vi "Read Controls from Config File.vi"(6 "Child?":bool, 7 "section":string, 8 "Error In":errorcluster, 9 "ParentName":string, 10 "Ctl Refnum":refnum<vi>, 11 "refnum":T1) -> (0 "Error Out":errorcluster, 3 "refnum out":T1)   [LabVIEW 2018]
uses:
  <vilib>/Utility/config.llb/Config Data RefNum.ctl
  Hardware Mfg/Thorlabs Translation Stages/Controls/Translation Stage Cluster.ctl
  Controls/Translation Stage Types.ctl
  <vilib>/Utility/config.llb/Read Key (String).vi
  <vilib>/Utility/config.llb/Read Key (Boolean).vi
  <vilib>/Utility/config.llb/Read Key (Double).vi
  <vilib>/Utility/config.llb/Read Key (U32).vi
  <vilib>/Utility/config.llb/NI_LVConfig.lvlib
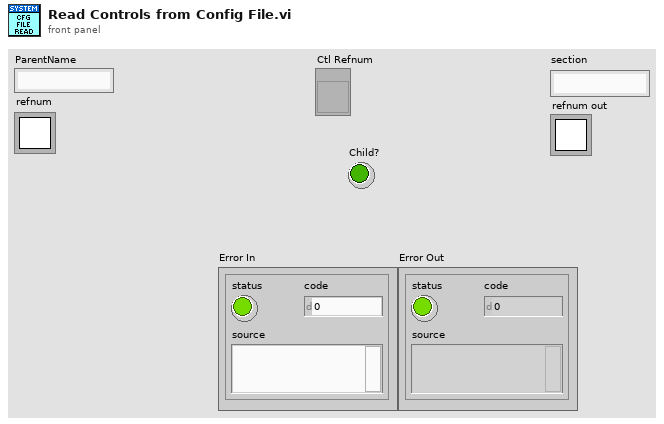
[diagram p1: front panel]
types:
  T1 = typedef "NI_LVConfig.lvlib/Config Data RefNum.ctl" = refnum<k1>
  T2 = typedef "Translation Stage Cluster.ctl" = cluster{"Position":dbl, "Is.Enabled?":bool, "Is.Connected?":bool, "Device SN":string, "AccelerationMaximum":dbl, "VelocityMaximum":dbl, "Acceleration":dbl, "Velocity":dbl, "waitTimeout (ms)":i32, "Model":T3, "Is.Homed?":bool, "MOVE":bool}
  T3 = typedef "Translation Stage Types.ctl" = enum16{"None", "Thorlabs LTS", "Thorlabs MLJ"}
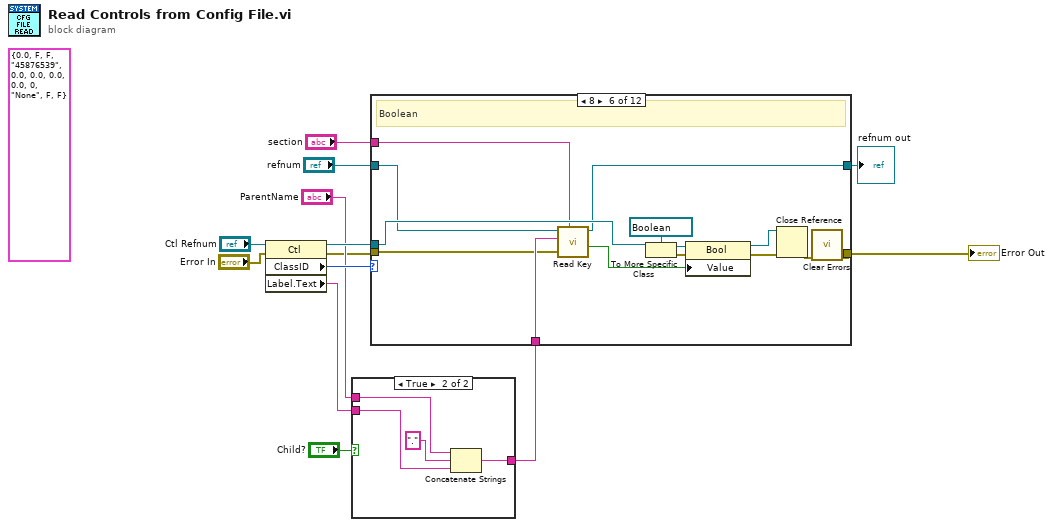
[diagram p0: block diagram]
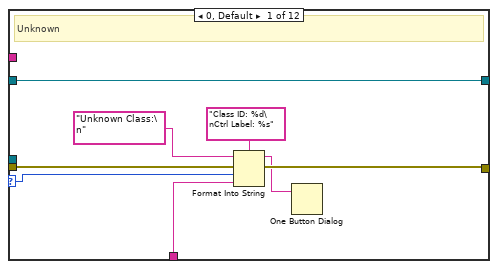
[diagram p3: hidden frame]
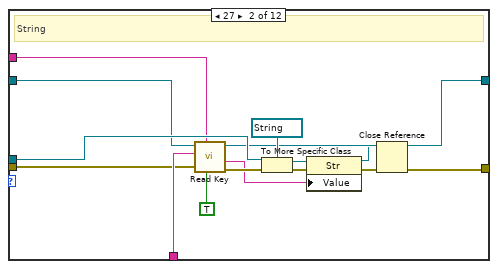
[diagram p4: hidden frame]
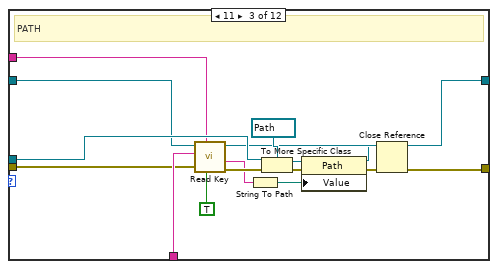
[diagram p5: hidden frame]
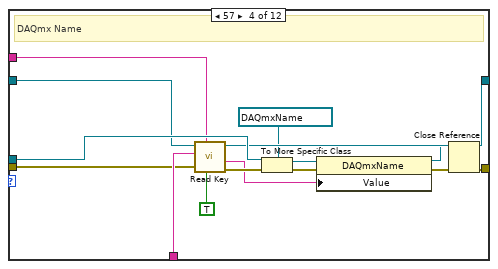
[diagram p6: hidden frame]
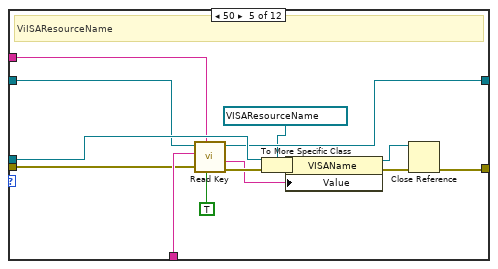
[diagram p7: hidden frame]
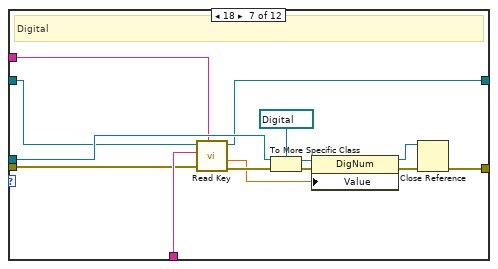
[diagram p8: hidden frame]
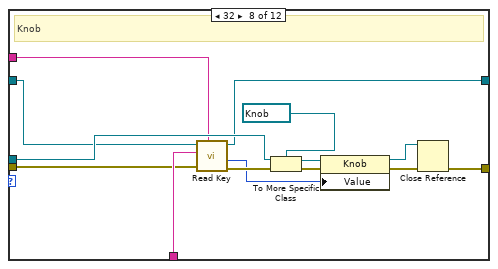
[diagram p9: hidden frame]
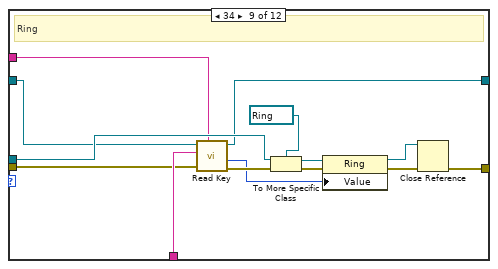
[diagram p10: hidden frame]
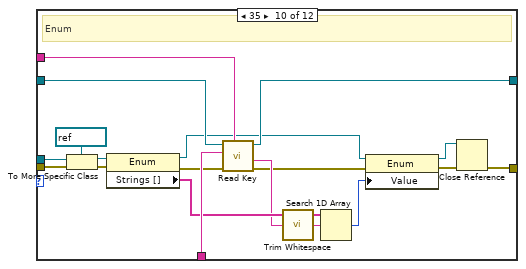
[diagram p11: hidden frame]
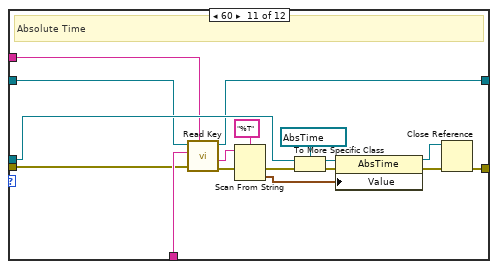
[diagram p12: hidden frame]
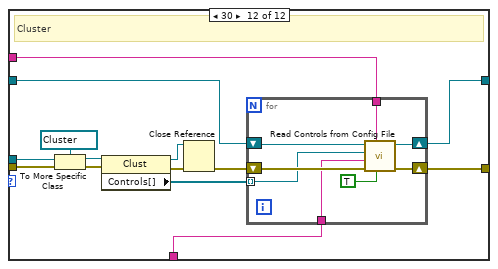
[diagram p13: hidden frame]
diagram:
  (unwired) T2 {"Position"=0.0, "Is.Enabled?"=FALSE, "Is.Connected?"=FALSE, "Device SN"="45876539", "AccelerationMaximum"=0.0, "VelocityMaximum"=0.0, "Acceleration"=0.0, "Velocity"=0.0, "waitTimeout (ms)"=0, "Model"=enum."None", "Is.Homed?"=FALSE, "MOVE"=FALSE} ("Control Param In")
  n1 = property class="Ctl"(reference="Ctl Refnum", error in="Error In") -> (reference out=w12:refnum<vi>, error out=w6:errorcluster, "ClassID"=w11:u32, "Label.Text"=w8:string)
  n2 = case shown="True" "Child?" {
    tunnel: "ParentName" -> [_ w18]
    tunnel: w8 -> [w14 w16]
    tunnel: [w14 w15] -> w3
    frame False {
    }
    frame True {
      n3 = Concatenate Strings(w18, ".", w16) -> (w15:string)
    }
  }
  n4 = case shown="8" w11 {
    selector: w11 -> [w23 _ _ _ _ _ _ _ _ _ _ _]
    tunnel: w6 -> [w21 w30 w46 w62 w77 w91 w104 w119 w133 w162 w168 w193]
    tunnel: w12 -> [_ w40 w56 w72 w87 w100 w115 w129 w143 w161 w179 w191]
    tunnel: [w20 w28 w44 w60 w75 w88 w105 w120 w134 w145 w169 w187] -> w1
    tunnel: "section" -> [_ w39 w55 w71 w86 w99 w108 w123 w137 w157 w173 w184]
    tunnel: "refnum" -> [w26 w38 w54 w70 w85 w98 w107 w122 w136 w156 w172 w186]
    tunnel: [w26 w37 w53 w69 w84 w97 w106 w121 w135 w155 w171 w185] -> w2
    tunnel: w3 -> [w22 w35 w51 w67 w82 w95 w109 w124 w138 w158 w174 w183]
    frame 0, Default {
      # "Unknown"
      n5 = Format Into String(format string="Class ID: %d\nCtrl Label: %s", initial string="Unknown Class:\n" ("string"), error in=w21, w23, w22) -> (resulting string=w19:string, error out=w20:errorcluster)
      n6 = One Button Dialog(message=w19) -> ()  [unwired: 1 in, 1 out]
    }
    frame 27 {
      # "String"
      n7 = call-poly <vilib>:"Read Key.vi"("read raw string? (F)"=TRUE, "section"=w39, "error in (no error)"=w30, "key"=w35, "refnum"=w38) -> ("error out"=w29:errorcluster, "value"=w27:string, "refnum out"=w37:T1)  [unwired: 3 in, 1 out]
      n8 = To More Specific Class(target class=refnum<vi> refnum ("AccelerationMaximum 2"), reference=w40, error in=w29) -> (specific class reference=w33:refnum<vi>, error out=w36:errorcluster)
      n9 = property class="Str"(reference=w33, error in=w36, "Value"=w27) -> (reference out=w32:refnum<vi>, error out=w34:errorcluster)
      n10 = Close Reference(reference=w32, error in (no error)=w34) -> (error out=w28:errorcluster)
    }
    frame 11 {
      # "PATH"
      n11 = call-poly <vilib>:"Read Key.vi"("read raw string? (F)"=TRUE, "section"=w55, "error in (no error)"=w46, "key"=w51, "refnum"=w54) -> ("error out"=w45:errorcluster, "value"=w43:string, "refnum out"=w53:T1)  [unwired: 3 in, 1 out]
      n12 = String To Path(string=w43) -> (path=w42:path)
      n13 = To More Specific Class(target class=refnum<vi> refnum ("AccelerationMaximum 2"), reference=w56, error in=w45) -> (specific class reference=w49:refnum<vi>, error out=w52:errorcluster)
      n14 = property class="Path"(reference=w49, error in=w52, "Value"=w42) -> (reference out=w48:refnum<vi>, error out=w50:errorcluster)
      n15 = Close Reference(reference=w48, error in (no error)=w50) -> (error out=w44:errorcluster)
    }
    frame 57 {
      # "DAQmx Name"
      n16 = call-poly <vilib>:"Read Key.vi"("read raw string? (F)"=TRUE, "section"=w71, "error in (no error)"=w62, "key"=w67, "refnum"=w70) -> ("error out"=w61:errorcluster, "value"=w59:string, "refnum out"=w69:T1)  [unwired: 3 in, 1 out]
      n17 = To More Specific Class(target class=refnum<vi> refnum ("Analog Out Channel"), reference=w72, error in=w61) -> (specific class reference=w65:refnum<vi>, error out=w68:errorcluster)
      n18 = property class="DAQmxName"(reference=w65, error in=w68, "Value"=w59) -> (reference out=w64:refnum<vi>, error out=w66:errorcluster)
      n19 = Close Reference(reference=w64, error in (no error)=w66) -> (error out=w60:errorcluster)
    }
    frame 50 {
      # "ViISAResourceName"
      n20 = call-poly <vilib>:"Read Key.vi"("read raw string? (F)"=TRUE, "section"=w86, "error in (no error)"=w77, "key"=w82, "refnum"=w85) -> ("error out"=w76:errorcluster, "value"=w74:string, "refnum out"=w84:T1)  [unwired: 3 in, 1 out]
      n21 = To More Specific Class(target class=refnum<vi> refnum ("Controller VISA Ref"), reference=w87, error in=w76) -> (specific class reference=w80:refnum<vi>, error out=w83:errorcluster)
      n22 = property class="VISAName"(reference=w80, error in=w83, "Value"=w74) -> (reference out=w79:refnum<vi>, error out=w81:errorcluster)
      n23 = Close Reference(reference=w79, error in (no error)=w81) -> (error out=w75:errorcluster)
    }
    frame 8 {
      # "Boolean"
      n24 = call-poly <vilib>:"Read Key.vi"("section"=w99, "error in (no error)"=w91, "key"=w95, "refnum"=w98) -> ("value"=w90:bool, "refnum out"=w97:T1)  [unwired: 4 in, 2 out]
      n25 = To More Specific Class(target class=refnum<vi> refnum ("AccelerationMaximum 2"), reference=w100) -> (specific class reference=w93:refnum<vi>, error out=w96:errorcluster)  [unwired: 1 in]
      n26 = property class="Bool"(reference=w93, error in=w96, "Value"=w90) -> (reference out=w92:refnum<vi>, error out=w94:errorcluster)
      n27 = Close Reference(reference=w92, error in (no error)=w94) -> (error out=w89:errorcluster)
      n28 = call <vilib>:"Clear Errors.vi"("error in (no error)"=w89) -> ("error out"=w88:errorcluster)  [unwired: 5 in, 1 out]
    }
    frame 18 {
      # "Digital"
      n29 = call-poly <vilib>:"Read Key.vi"("section"=w108, "error in (no error)"=w104, "key"=w109, "refnum"=w107) -> ("error out"=w103:errorcluster, "value"=w102:dbl, "refnum out"=w106:T1)  [unwired: 4 in, 1 out]
      n30 = To More Specific Class(target class=refnum<vi> refnum ("AccelerationMaximum 2"), reference=w115, error in=w103) -> (specific class reference=w112:refnum<vi>, error out=w113:errorcluster)
      n31 = property class="DigNum"(reference=w112, error in=w113, "Value"=w102) -> (reference out=w110:refnum<vi>, error out=w111:errorcluster)
      n32 = Close Reference(reference=w110, error in (no error)=w111) -> (error out=w105:errorcluster)
    }
    frame 32 {
      # "Knob"
      n33 = call-poly <vilib>:"Read Key.vi"("section"=w123, "error in (no error)"=w119, "key"=w124, "refnum"=w122) -> ("error out"=w118:errorcluster, "value"=w117:u32, "refnum out"=w121:T1)  [unwired: 4 in, 1 out]
      n34 = To More Specific Class(target class=refnum<vi> refnum ("Zoom Factor"), reference=w129, error in=w118) -> (specific class reference=w127:refnum<vi>, error out=w128:errorcluster)
      n35 = property class="Knob"(reference=w127, error in=w128, "Value"=w117) -> (reference out=w125:refnum<vi>, error out=w126:errorcluster)
      n36 = Close Reference(reference=w125, error in (no error)=w126) -> (error out=w120:errorcluster)
    }
    frame 34 {
      # "Ring"
      n37 = call-poly <vilib>:"Read Key.vi"("section"=w137, "error in (no error)"=w133, "key"=w138, "refnum"=w136) -> ("error out"=w132:errorcluster, "value"=w131:u32, "refnum out"=w135:T1)  [unwired: 4 in, 1 out]
      n38 = To More Specific Class(target class=refnum<vi> refnum ("Trigger Operation"), reference=w143, error in=w132) -> (specific class reference=w141:refnum<vi>, error out=w142:errorcluster)
      n39 = property class="Ring"(reference=w141, error in=w142, "Value"=w131) -> (reference out=w139:refnum<vi>, error out=w140:errorcluster)
      n40 = Close Reference(reference=w139, error in (no error)=w140) -> (error out=w134:errorcluster)
    }
    frame 35 {
      # "Enum"
      n41 = To More Specific Class(target class=refnum<vi> refnum ("Enum"), reference=w161, error in=w162) -> (specific class reference=w159:refnum<vi>, error out=w160:errorcluster)
      n42 = property class="Enum"(reference=w159, error in=w160) -> (reference out=w146:refnum<vi>, error out=w152:errorcluster, "Strings []"=w153:string[])
      n43 = call-poly <vilib>:"Read Key.vi"("section"=w157, "error in (no error)"=w152, "key"=w158, "refnum"=w156) -> ("error out"=w150:errorcluster, "value"=w151:string, "refnum out"=w155:T1)  [unwired: 4 in, 1 out]
      n44 = call <vilib>:"Trim Whitespace.vi"("string"=w151) -> ("trimmed string"=w148:string)  [unwired: 1 in]
      n45 = Search 1D Array(1D array=w153, element=w148) -> (index of element=w147:i32)  [unwired: 1 in]
      n46 = property class="Enum"(reference=w146, error in=w150, "Value"=w147) -> (reference out=w144:refnum<vi>, error out=w149:errorcluster)
      n47 = Close Reference(reference=w144, error in (no error)=w149) -> (error out=w145:errorcluster)
    }
    frame 60 {
      # "Absolute Time"
      n48 = call-poly <vilib>:"Read Key.vi"("section"=w173, "error in (no error)"=w168, "key"=w174, "refnum"=w172) -> ("error out"=w166:errorcluster, "value"=w163:string, "refnum out"=w171:T1)  [unwired: 4 in, 1 out]
      n49 = Scan From String(format string="%T", input string=w163, error in=w166) -> (error out=w165:errorcluster, output 1=w164:timestamp)  [unwired: 2 in, 2 out]
      n50 = To More Specific Class(target class=refnum<vi> refnum ("AccelerationMaximum 2"), reference=w179, error in=w165) -> (specific class reference=w177:refnum<vi>, error out=w178:errorcluster)
      n51 = property class="AbsTime"(reference=w177, error in=w178, "Value"=w164) -> (reference out=w175:refnum<vi>, error out=w176:errorcluster)
      n52 = Close Reference(reference=w175, error in (no error)=w176) -> (error out=w169:errorcluster)
    }
    frame 30 {
      # "Cluster"
      n53 = To More Specific Class(target class=refnum<vi> refnum ("Cluster Ref In"), reference=w191, error in=w193) -> (specific class reference=w189:refnum<vi>, error out=w190:errorcluster)
      n54 = property class="Clust"(reference=w189, error in=w190) -> (reference out=w181:refnum<vi>, error out=w188:errorcluster, "Controls[]"=w180:refnum<vi>[])
      n55 = Close Reference(reference=w181, error in (no error)=w188) -> (error out=w182:errorcluster)
      n56 = for {
        tunnel: w184 -> [w197]
        tunnel: w183 -> [w196]
        shift-right: [w200] -> w187
        shift-left: w182 -> [w201]
        shift-right: [w198] -> w185
        shift-left: w186 -> [w199]
        tunnel: w180 -> [w194] mode=indexing
        n57 = call "Read Controls from Config File.vi"("Child?"=TRUE, "section"=w197, "Error In"=w201, "ParentName"=w196, "Ctl Refnum"=w194, "refnum"=w199) -> ("Error Out"=w200:errorcluster, "refnum out"=w198:T1)  [unwired: 4 in]
      }
    }
  }
  "Error Out" <- w1
  "refnum out" <- w2
